vi "FTW-Producer-Destroy.vi"(0 "FTW-Producer In":refnum<class "FTW-Producer.lvclass">, 11 "error in":errorcluster) -> (15 "error out":errorcluster)   [LabVIEW 2015, in "FTW-Producer.lvclass"]
uses:
  FTW-Producer.lvclass
  FTW-Producer.lvclass/FTW-Producer.ctl
  Endpoint/FTW-Endpoint.lvclass
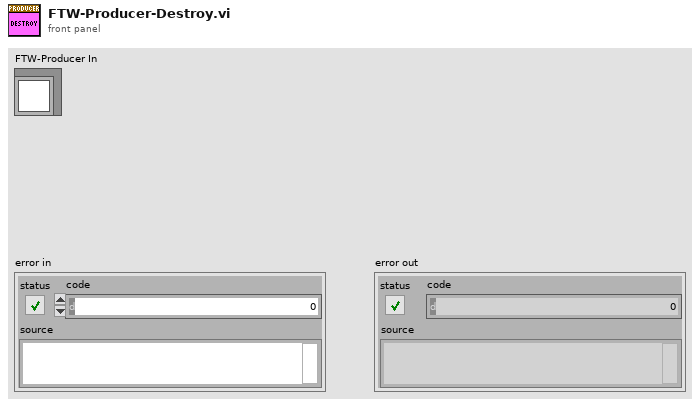
[diagram p1: front panel]
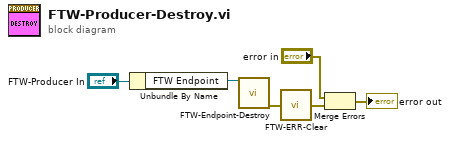
[diagram p0: block diagram]
diagram:
  n1 = Unbundle By Name("FTW-Producer In") -> ("FTW Endpoint"=w3:refnum<class "FTW-Endpoint.lvclass">)
  n2 = call-dynamic "FTW-Endpoint-Destroy.vi"("FTW Endpoint"=w3) -> ("error out"=w2:errorcluster)  [unwired: 14 in]
  n3 = call "FTW-ERR-Clear.vi"("error to snuff"=w2) -> ("no error"=w1:errorcluster)
  n4 = Merge Errors("error in", w1) -> (→"error out":errorcluster)
